vi "Forward Dynamics.vi"(5 "data":variant, 6 "simulation parameters":T2={"Initial Time"=0.0, "Final Time"=10.0, "Time Step"=0.1, "Absolute Tolerance"=0.001, "Relative Tolerance"=0.001, "Continuous Solver"=enum."Runge-Kutta 45 (variable)", "Discrete Time Step"=1.0, "Minimum Time Step"=1e-08, "Maximum Time Step"=1.0, "Initial Time Step"=0.01} {"Initial Time Step" min=0.0; "Maximum Time Step" min=0.0; "Absolute Tolerance" format="%#_6f"}, 7 "torque function":refnum<vi>, 8 "error in (no error)":errorcluster, 10 "integration data":T1, 11 "serial arm in":refnum<class "NI_Robotics_Serial Robot Arm.lvclass">) -> (0 "error out":errorcluster, 1 "joint velocity trajectory":dbl[][](array[numeric]), 2 "joint position trajectory":dbl[][](array[numeric]), 3 "serial arm out":refnum<class "NI_Robotics_Serial Robot Arm.lvclass">, 4 "times":dbl[](array[numeric]))   [LabVIEW 2017, in "NI_Kinematics.lvlib"]
doc: "Computes the joint angles and movements of a robot arm that result from applying a given amount of torque to the arm over a period of time.\n\n<B>.m file:</B> fdyn"
uses:
  <vilib>/robotics/Kinematics/NI_Kinematics.lvlib
  <vilib>/robotics/Kinematics/Robot/NI_Robotics_Serial Robot Arm.lvclass
  <vilib>/Simulation/Utility/Implementation/Shared/SIM Diagram Parameters.ctl
  <vilib>/Simulation/Implementation/Shared/SIM Continuous Solvers.ctl
  <vilib>/robotics/Kinematics/dyn/fdyn_helper_data.ctl
  <vilib>/gmath/ode.llb/ODE Solver main.vi
  <vilib>/gmath/NI_Gmath.lvlib
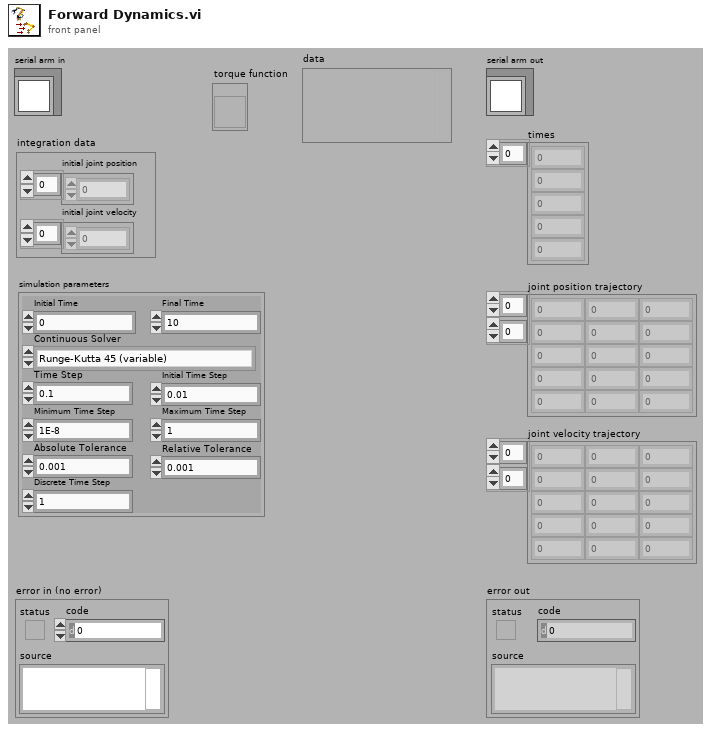
[diagram p1: front panel]
types:
  T1 = cluster{"initial joint position":dbl[], "initial joint velocity":dbl[]}
  T2 = typedef "SIM Diagram Parameters.ctl" = cluster{"Initial Time":dbl, "Final Time":dbl, "Time Step":dbl, "Absolute Tolerance":dbl, "Relative Tolerance":dbl, "Continuous Solver":T3, "Discrete Time Step":dbl, "Minimum Time Step":dbl, "Maximum Time Step":dbl, "Initial Time Step":dbl}
  T3 = typedef "SIM Continuous Solvers.ctl" = enum16{"Runge-Kutta 1 (Euler)", "Runge-Kutta 2", "Runge-Kutta 3", "Runge-Kutta 4", "Runge-Kutta 23 (variable)", "Runge-Kutta 45 (variable)", "BDF (variable)", "Adams-Moulton (variable)", "Rosenbrock (variable)", "Discrete States Only"}
  T4 = typedef "NI_Kinematics.lvlib/fdyn_helper_data.ctl" = cluster{"Robot In":refnum<class "NI_Robotics_Serial Robot Arm.lvclass">, "Torque Function":refnum<vi>, "Torque Function Data":variant}
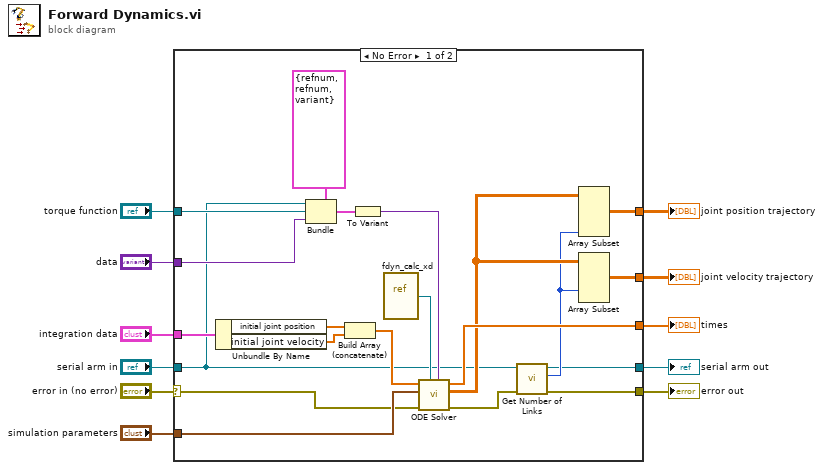
[diagram p0: block diagram]
diagram:
  n1 = case shown="No Error" "error in (no error)" {
    selector: "error in (no error)" -> [w12 w34]
    tunnel: [w31 _] -> w11
    tunnel: "torque function" -> [w30 _]
    tunnel: "data" -> [w29 _]
    tunnel: [w24 _] -> w8
    tunnel: [w23 _] -> w7
    tunnel: "integration data" -> [w22 _]
    tunnel: [w16 w34] -> w5
    tunnel: "serial arm in" -> [w15 w33]
    tunnel: [w14 w33] -> w3
    tunnel: "simulation parameters" -> [w13 _]
    frame No Error {
      n2 = Unbundle By Name(w22) -> ("initial joint position"=w20:dbl[], "initial joint velocity"=w21:dbl[])
      n3 = Bundle(cluster=T4 {"Robot In"=refnum, "Torque Function"=refnum, "Torque Function Data"=variant} ("fdyn_helper_data"), "Robot In"=w15, "Torque Function"=w30, "Torque Function Data"=w29) -> (w28:T4)
      n4 = Build Array (concatenate)(w20, w21) -> (w32:dbl[])
      n5 = To Variant(anything=w28) -> (Variant=w27:variant)
      n6 = vi-ref <vilib>:"fdyn_calc_xd.vi"() -> (w26:refnum<vi>)
      n7 = call-poly <vilib>:"ODE Solver.vi"("data"=w27, "ODE F(X,t)"=w26, "error in (no error)"=w12, "simulation parameters"=w13, "x0"=w32) -> ("error out"=w17:errorcluster, "outputs"=w25:dbl[][], "times"=w31:dbl[])  [unwired: 4 in]
      n8 = call <vilib>:"Get Number of Links.vi"("error in (no error)"=w17, "serial arm in"=w15) -> ("error out"=w16:errorcluster, "number of links"=w19:i32, "serial arm out"=w14:refnum<class "NI_Robotics_Serial Robot Arm.lvclass">)  [unwired: 7 in]
      n9 = Array Subset(array=w25, length (col)=w19) -> (w23:dbl[][])  [unwired: 3 in]
      n10 = Array Subset(array=w25, index (col)=w19) -> (w24:dbl[][])  [unwired: 3 in]
    }
    frame Error {
    }
  }
  "serial arm out" <- w3
  "joint position trajectory" <- w7
  "times" <- w11
  "joint velocity trajectory" <- w8
  "error out" <- w5
